vi "Null treatment.vi"() -> ()   [LabVIEW 2017]
uses:
  c739188d-e448-4d63-9b92-24f3593d0701.vi
  JSONtext.lvlib
  <vilib>/addons/_JKI Toolkits/Caraya/classes/Assert/Assert.lvclass
  <vilib>/addons/_JKI Toolkits/Caraya/classes/Test/Test.lvclass
panel:
  out "error out":errorcluster
  out "Array 4":T1(array[cluster])
  out "Array 3":i32[](array[numeric])
  # "See Issue #65"
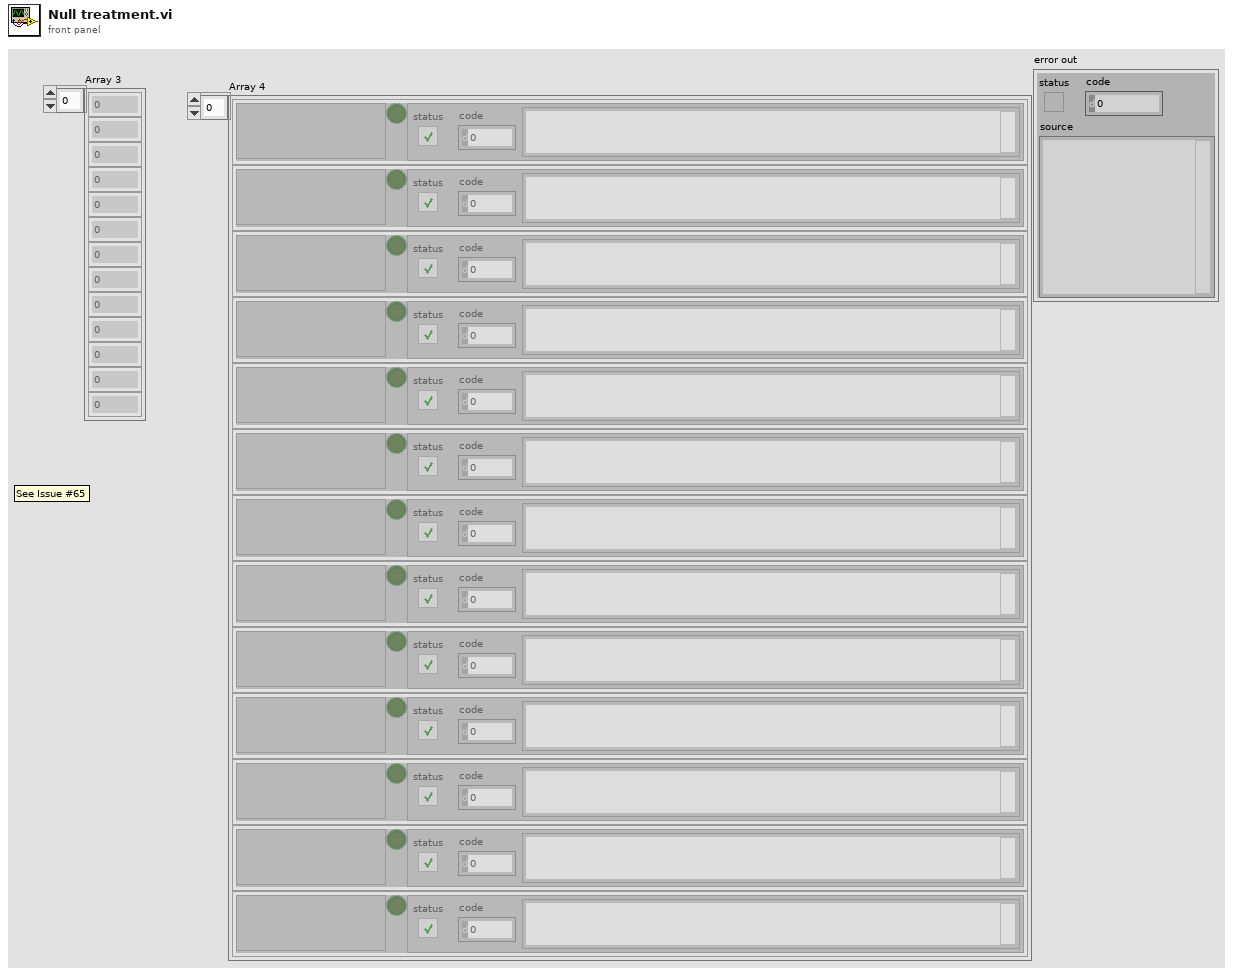
[diagram p1: front panel]
types:
  T1 = cluster{"Variant out":variant, bool, "error out":errorcluster}[]
  T2 = cluster{"Variant out":variant, bool, "error out":errorcluster}
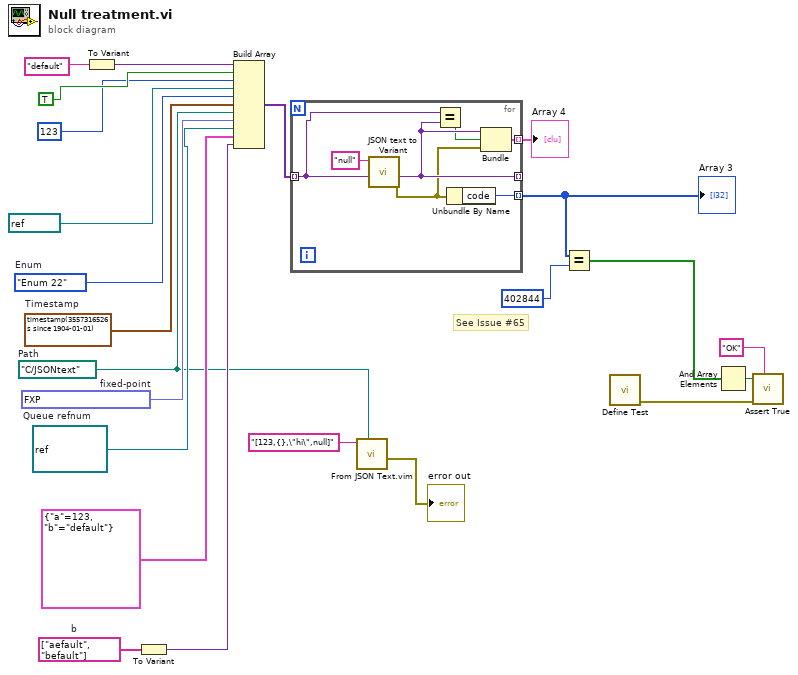
[diagram p0: block diagram]
diagram:
  w10 = string[] ["aefault", "befault"]  # b
  w16 = timestamp(3557316526.864 s since 1904-01-01)  # Timestamp
  w15 = refnum<queue> refnum  # Queue refnum
  w7 = path "C:/JSONtext"  # Path
  w13 = fxp<+/-,32,16> 32767.899993896484  # fixed-point
  w17 = enum16{"Enum 1", "Enum 22", "Enum 333"}."Enum 22"  # Enum
  # "See Issue #65"
  n1 = To Variant(anything="default") -> (Variant=w22:variant)
  n2 = To Variant(anything=w10) -> (Variant=w11:variant)
  n3 = Build Array(w22, TRUE, 123, refnum<visa-resource-name> "com" ("VISA resource name"), w17, w16, w7, w13, w15, cluster{"a":i32, "b":string} {"a"=123, "b"="default"}, w11) -> (w19:variant[])
  n4 = for {
    tunnel: w19 -> [w27] mode=indexing
    tunnel: [w28] -> _ mode=indexing
    tunnel: [w29] -> w3 mode=indexing
    tunnel: [w24] -> w9 mode=indexing
    n5 = call "JSON text to Variant.vi"("Data Type"=w27, "JSON"="null") -> ("error out"=w25:errorcluster, "Variant out"=w28:variant)  [unwired: 8 in]
    n6 = Equal?(x=w27, y=w28) -> (x = y?=w26:bool)
    n7 = Unbundle By Name(w25) -> ("code"=w29:i32)
    n8 = Bundle("Variant out"=w28, w26, "error out"=w25) -> (w24:T2)  [unwired: 1 in]
  }
  "Array 3" <- w3
  "Array 4" <- w9
  n9 = call "From JSON Text.vim"("Data Type and Default Value"=w7, "JSON"="[123,{},\"hi\",null]") -> ("error out"=→"error out":errorcluster)  [unwired: 8 in, 1 out]
  n10 = Equal?(x=w3, y=402844 ("code")) -> (x = y?=w1:bool[])
  n11 = call <vilib>:"Define Test.vi"() -> ("error out"=w4:errorcluster)  [unwired: 11 in]
  n12 = And Array Elements(Boolean array=w1) -> (logical AND=w6:bool)
  n13 = call <vilib>:"Assert True.vi"("Label"="OK", "error in (no error)"=w4, "True?"=w6) -> ()  [unwired: 8 in, 1 out]
